vi "Load Becker-Hickl Measurement Histo Information.vi"(8 "error in (no error)":errorcluster, 10 "Measurement FCS Info in":T1, 11 "string in":string) -> (0 "error out":errorcluster, 2 "Measurement FCS Info out":T1, 3 "string out":string)   [LabVIEW 2021, in "Becker-Hickl Files.lvlib"]
uses:
  Becker-Hickl Files.lvlib
  Becker-Hickl Additional Histogram Measurement Info.ctl
  Becker-Hickl Read Single SGL.vi
  Becker-Hickl Read Single I32.vi
  Becker-Hickl Read Single U32.vi
  Becker-Hickl Read Single DBL.vi
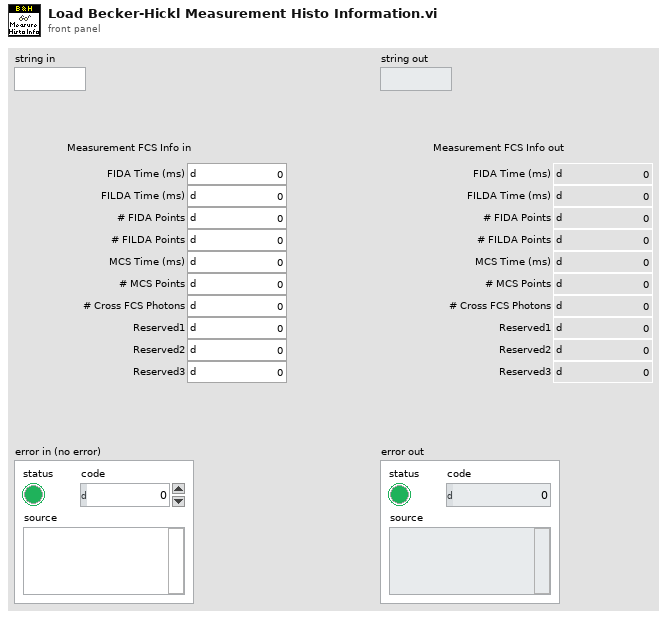
[diagram p1: front panel]
types:
  T1 = typedef "Becker-Hickl Files.lvlib/Becker-Hickl Additional Histogram Measurement Info.ctl" = cluster{"FIDA Time (ms)":sgl, "FILDA Time (ms)":sgl, "# FIDA Points":i32, "# FILDA Points":i32, "MCS Time (ms)":sgl, "# MCS Points":i32, "# Cross FCS Photons":u32, "Reserved1":i32, "Reserved2":dbl, "Reserved3":dbl}
  T2 = enum16{"fida_time", "filda_time", "fida_points", "filda_points", "mcs_time", "mcs_points", "cross_calc_phot", "reserved1", "reserved2", "reserved3"}
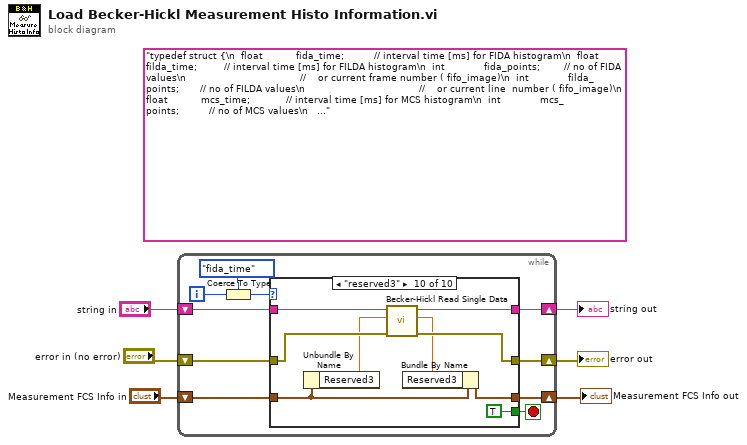
[diagram p0: block diagram]
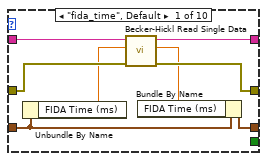
[diagram p2: hidden frame]
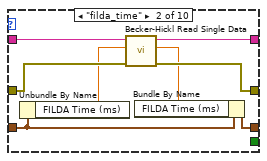
[diagram p3: hidden frame]
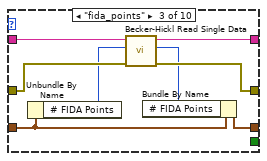
[diagram p4: hidden frame]
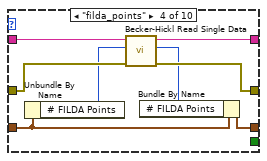
[diagram p5: hidden frame]
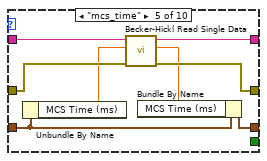
[diagram p6: hidden frame]
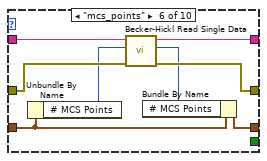
[diagram p7: hidden frame]
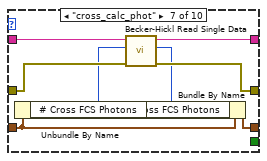
[diagram p8: hidden frame]
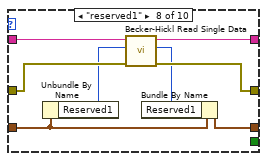
[diagram p9: hidden frame]
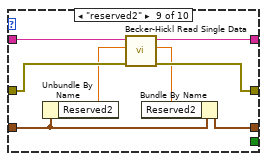
[diagram p10: hidden frame]
diagram:
  (unwired) "typedef struct {\n  float           fida_time;          // interval time [ms] for FIDA histogram\n  float           filda_time;         // interval time [ms] for FILDA histogram\n  int             fida_points;        // no of FIDA values\n                                      //    or current frame number ( fifo_image)\n  int             filda_points;       // no of FILDA values\n                                      //    or current line  number ( fifo_image)\n  float           mcs_time;            // interval time [ms] for MCS histogram\n  int             mcs_points;          // no of MCS values\n                                      //    or current pixel number ( fifo_image)\n  unsigned int    cross_calc_phot;    //  no of calculated photons from cross_channel \n                                      //    for Cross FCS histogram\n  int             reserved1;\n  double          reserved2;\n  double          reserved3;\n  }MeasHISTInfo;     // extension of MeasFCSInfo for other histograms ( FIDA, FILDA, MCS ) \n  \n"
  n1 = while {
    shift-right: [w12] -> w5
    shift-left: "string in" -> [w15]
    shift-right: [w11] -> w3
    shift-left: "error in (no error)" -> [w14]
    shift-right: [w10] -> w1
    shift-left: "Measurement FCS Info in" -> [w13]
    i -> [w16]
    stop <- w7 stop-if-true
    n2 = Coerce To Type(0:w16, 1:T2."fida_time") -> (2:w9:T2)
    n3 = case shown="\"reserved3\"" w9 {
      tunnel: w15 -> [w24 w32 w40 w48 w56 w64 w72 w80 w88 w97]
      tunnel: w14 -> [w21 w29 w37 w45 w53 w61 w69 w77 w85 w94]
      tunnel: w13 -> [w20 w28 w36 w44 w52 w60 w68 w76 w84 w93]
      tunnel: [w23 w31 w39 w47 w55 w63 w71 w79 w87 w96] -> w12
      tunnel: [w22 w30 w38 w46 w54 w62 w70 w78 w86 w95] -> w11
      tunnel: [w18 w26 w34 w42 w50 w58 w66 w74 w82 w91] -> w10
      tunnel: [_ _ _ _ _ _ _ _ _ TRUE] -> w7
      frame "fida_time", Default {
        n4 = Unbundle By Name(w20) -> ("FIDA Time (ms)"=w19:sgl)
        n5 = call-poly "Becker-Hickl Read Single Data.vi"("Error In"=w21, "Default"=w19, "Bytes in"=w24) -> ("Error Out"=w22:errorcluster, "SGL"=w17:sgl, "Bytes out"=w23:string)  [unwired: 6 in]
        n6 = Bundle By Name(cluster=w20, "FIDA Time (ms)"=w17) -> (w18:T1)
      }
      frame "filda_time" {
        n7 = Unbundle By Name(w28) -> ("FILDA Time (ms)"=w27:sgl)
        n8 = call-poly "Becker-Hickl Read Single Data.vi"("Error In"=w29, "Default"=w27, "Bytes in"=w32) -> ("Error Out"=w30:errorcluster, "SGL"=w25:sgl, "Bytes out"=w31:string)  [unwired: 6 in]
        n9 = Bundle By Name(cluster=w28, "FILDA Time (ms)"=w25) -> (w26:T1)
      }
      frame "fida_points" {
        n10 = Unbundle By Name(w36) -> ("# FIDA Points"=w35:i32)
        n11 = call-poly "Becker-Hickl Read Single Data.vi"("Error In"=w37, "Default"=w35, "Bytes in"=w40) -> ("Error Out"=w38:errorcluster, "I32"=w33:i32, "Bytes out"=w39:string)  [unwired: 6 in]
        n12 = Bundle By Name(cluster=w36, "# FIDA Points"=w33) -> (w34:T1)
      }
      frame "filda_points" {
        n13 = Unbundle By Name(w44) -> ("# FILDA Points"=w43:i32)
        n14 = call-poly "Becker-Hickl Read Single Data.vi"("Error In"=w45, "Default"=w43, "Bytes in"=w48) -> ("Error Out"=w46:errorcluster, "I32"=w41:i32, "Bytes out"=w47:string)  [unwired: 6 in]
        n15 = Bundle By Name(cluster=w44, "# FILDA Points"=w41) -> (w42:T1)
      }
      frame "mcs_time" {
        n16 = Unbundle By Name(w52) -> ("MCS Time (ms)"=w51:sgl)
        n17 = call-poly "Becker-Hickl Read Single Data.vi"("Error In"=w53, "Default"=w51, "Bytes in"=w56) -> ("Error Out"=w54:errorcluster, "SGL"=w49:sgl, "Bytes out"=w55:string)  [unwired: 6 in]
        n18 = Bundle By Name(cluster=w52, "MCS Time (ms)"=w49) -> (w50:T1)
      }
      frame "mcs_points" {
        n19 = Unbundle By Name(w60) -> ("# MCS Points"=w59:i32)
        n20 = call-poly "Becker-Hickl Read Single Data.vi"("Error In"=w61, "Default"=w59, "Bytes in"=w64) -> ("Error Out"=w62:errorcluster, "I32"=w57:i32, "Bytes out"=w63:string)  [unwired: 6 in]
        n21 = Bundle By Name(cluster=w60, "# MCS Points"=w57) -> (w58:T1)
      }
      frame "cross_calc_phot" {
        n22 = Unbundle By Name(w68) -> ("# Cross FCS Photons"=w67:u32)
        n23 = call-poly "Becker-Hickl Read Single Data.vi"("Error In"=w69, "Default"=w67, "Bytes in"=w72) -> ("Error Out"=w70:errorcluster, "U32"=w65:u32, "Bytes out"=w71:string)  [unwired: 6 in]
        n24 = Bundle By Name(cluster=w68, "# Cross FCS Photons"=w65) -> (w66:T1)
      }
      frame "reserved1" {
        n25 = Unbundle By Name(w76) -> ("Reserved1"=w75:i32)
        n26 = call-poly "Becker-Hickl Read Single Data.vi"("Error In"=w77, "Default"=w75, "Bytes in"=w80) -> ("Error Out"=w78:errorcluster, "I32"=w73:i32, "Bytes out"=w79:string)  [unwired: 6 in]
        n27 = Bundle By Name(cluster=w76, "Reserved1"=w73) -> (w74:T1)
      }
      frame "reserved2" {
        n28 = Unbundle By Name(w84) -> ("Reserved2"=w83:dbl)
        n29 = call-poly "Becker-Hickl Read Single Data.vi"("Error In"=w85, "Default"=w83, "Bytes in"=w88) -> ("Error Out"=w86:errorcluster, "DBL"=w81:dbl, "Bytes out"=w87:string)  [unwired: 6 in]
        n30 = Bundle By Name(cluster=w84, "Reserved2"=w81) -> (w82:T1)
      }
      frame "reserved3" {
        n31 = Unbundle By Name(w93) -> ("Reserved3"=w92:dbl)
        n32 = call-poly "Becker-Hickl Read Single Data.vi"("Error In"=w94, "Default"=w92, "Bytes in"=w97) -> ("Error Out"=w95:errorcluster, "DBL"=w90:dbl, "Bytes out"=w96:string)  [unwired: 6 in]
        n33 = Bundle By Name(cluster=w93, "Reserved3"=w90) -> (w91:T1)
      }
    }
  }
  "Measurement FCS Info out" <- w1
  "error out" <- w3
  "string out" <- w5
